vi "MultiRun Status.vi"(1 "Input Array":string[](array[string])) -> (0 "Table Control":string[][](table))   [LabVIEW 2022 SP3]
uses:
  Globals/Trav_pos_global.vi
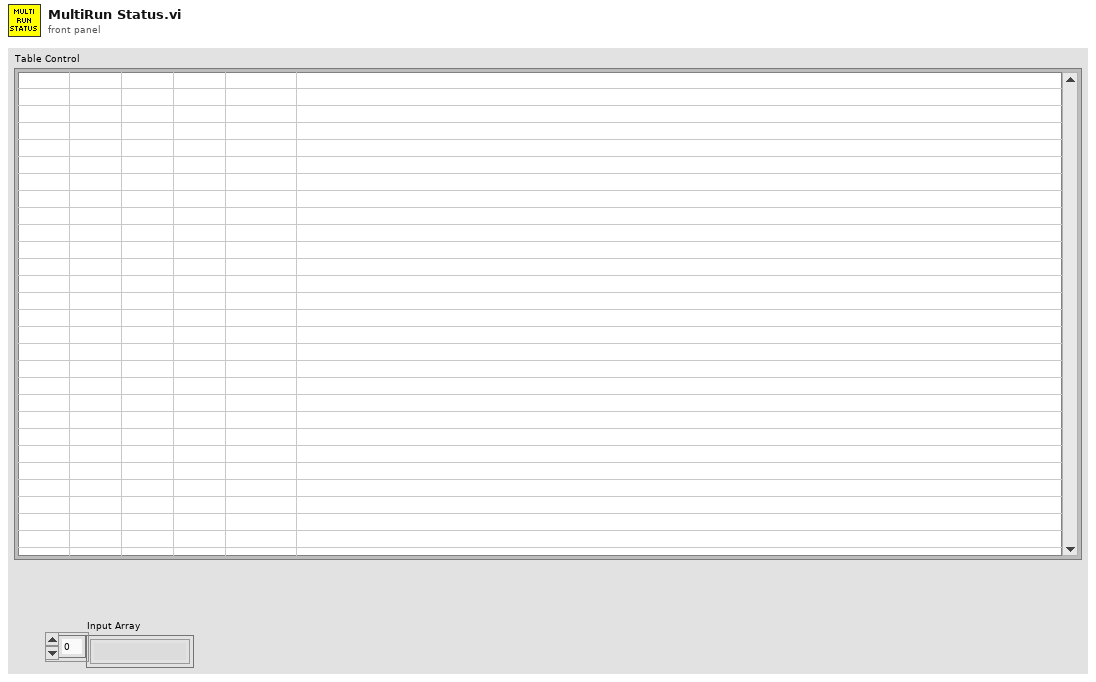
[diagram p1: front panel]
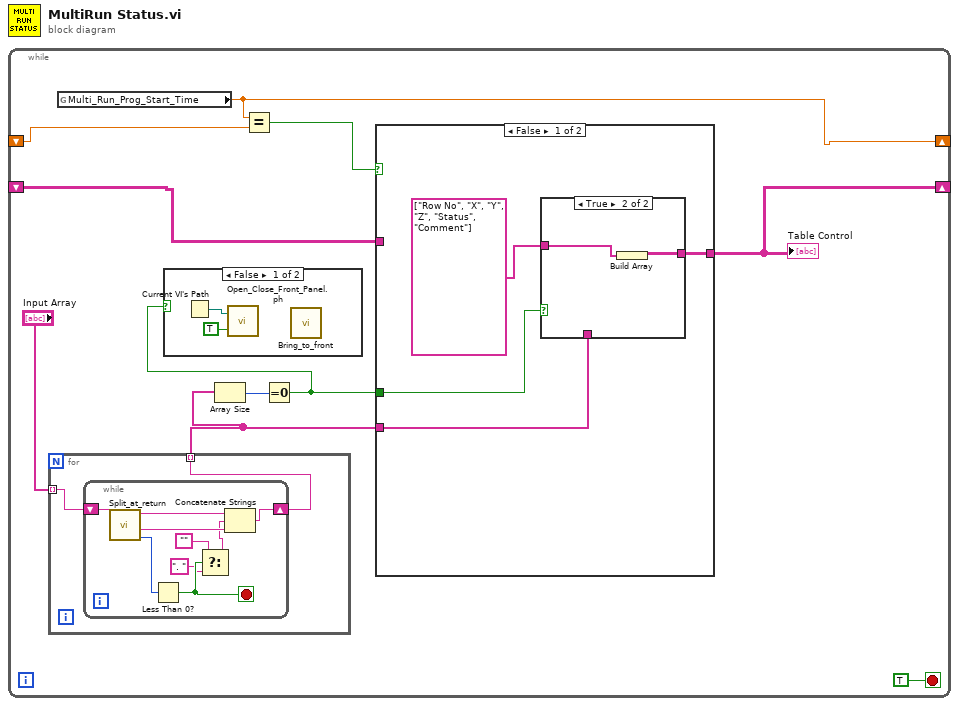
[diagram p0: block diagram]
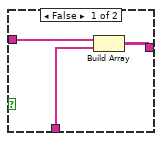
[diagram p3: hidden frame]
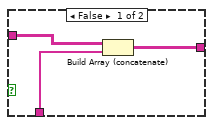
[diagram p5: hidden frame]
diagram:
  n1 = while {
    shift-right: [w8] -> _
    shift-left: _ -> [w9]
    shift-right: [w1] -> _
    shift-left: _ -> [w2]
    stop <- TRUE stop-if-true
    n2 = for {
      tunnel: "Input Array" -> [w14] mode=indexing
      tunnel: [w13] -> w4 mode=indexing
      n3 = while {
        shift-right: [w21] -> w13
        shift-left: w14 -> [w23]
        stop <- w18 stop-if-true
        n4 = call "Split_at_return.vi"("String"=w23) -> ("before substring"=w22:string, "after substring"=w19:string, "offset past match"=w20:i32)  [unwired: 1 in, 1 out]
        n5 = Less Than 0?(x=w20) -> (x < 0?=w18:bool)
        n6 = Select(t="", s=w18, f=". " ("string")) -> (s? t:f=w15:string)
        n7 = Concatenate Strings(w22, w15, w19) -> (w21:string)
      }
    }
    n8 = global read "Trav_pos_global.vi" "Multi_Run_Prog_Start_Time"() -> (w8:dbl)
    n9 = Array Size(array=w4) -> (size(s)=w6:i32)
    n10 = Equal?(x=w8, y=w9) -> (x = y?=w7:bool)
    n11 = Equal To 0?(x=w6) -> (x = 0?=w3:bool)
    n12 = case shown="False" w3 {
      frame False {
        n13 = Current VI's Path() -> (path=w11:path)
        n14 = call "Open_Close_Front_Panel.ph.vi"("openWindow (T)"=TRUE ("Front Panel Window:Open"), "VI path"=w11) -> ()  [unwired: 1 in, 1 out]
        n15 = call "Bring_to_front.vi"() -> ()  [unwired: 1 in]
      }
      frame True {
      }
    }
    n16 = case shown="False" w7 {
      tunnel: w2 -> [_ w36]
      tunnel: w4 -> [w27 w35]
      tunnel: [w26 w34] -> w1
      tunnel: w3 -> [w24 w33]
      frame False {
        n17 = case shown="True" w24 {
          tunnel: w27 -> [w30 _]
          tunnel: [w29 w31] -> w26
          tunnel: string[] ["Row No", "X", "Y", "Z", "Status", "Comment"] ("Jumped Positions") -> [w28 w32]
          frame False {
            n18 = Build Array(w28, w30) -> (w29:string[][])
          }
          frame True {
            n19 = Build Array(w32) -> (w31:string[][])
          }
        }
      }
      frame True {
        n20 = case shown="True" w33 {
          tunnel: w36 -> [w39 w40]
          tunnel: w35 -> [w38 _]
          tunnel: [w37 w40] -> w34
          frame False {
            n21 = Build Array (concatenate)(w39, w38) -> (w37:string[][])
          }
          frame True {
          }
        }
      }
    }
    "Table Control" <- w1
  }
